vi "CASE STRUCTURE WITH BOOLEAN.vi"() -> ()   [LabVIEW 2018]
panel:
  out "RESULT":dbl
  in  "Y":dbl
  in  "X":dbl
  in  "CS":bool
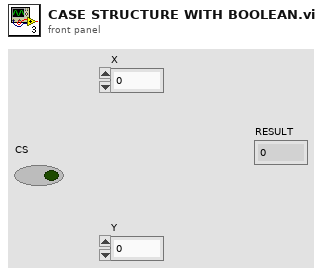
[diagram p1: front panel]
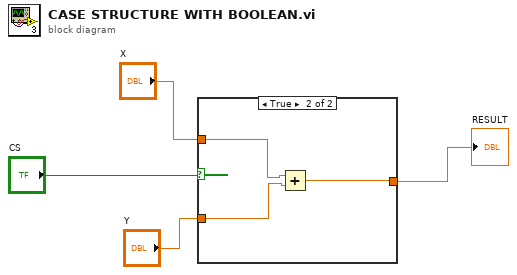
[diagram p0: block diagram]
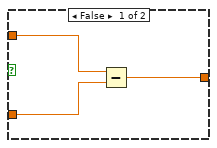
[diagram p2: hidden frame]
diagram:
  n1 = case shown="True" "CS" {
    tunnel: "X" -> [w7 w9]
    tunnel: "Y" -> [w6 w10]
    tunnel: [w5 w8] -> w1
    frame False {
      n2 = Subtract(x=w7, y=w6) -> (x-y=w5:dbl)
    }
    frame True {
      n3 = Add(x=w9, y=w10) -> (x+y=w8:dbl)
    }
  }
  "RESULT" <- w1
